vi "Display_ping.vi"(11 "Systèmes inatteignable":string[][](array[string])) -> ()   [LabVIEW 2019]
panel:
  in  "Bouton OK":bool
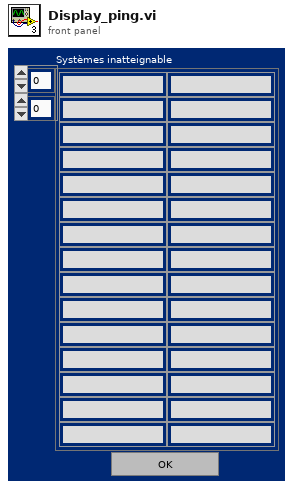
[diagram p1: front panel]
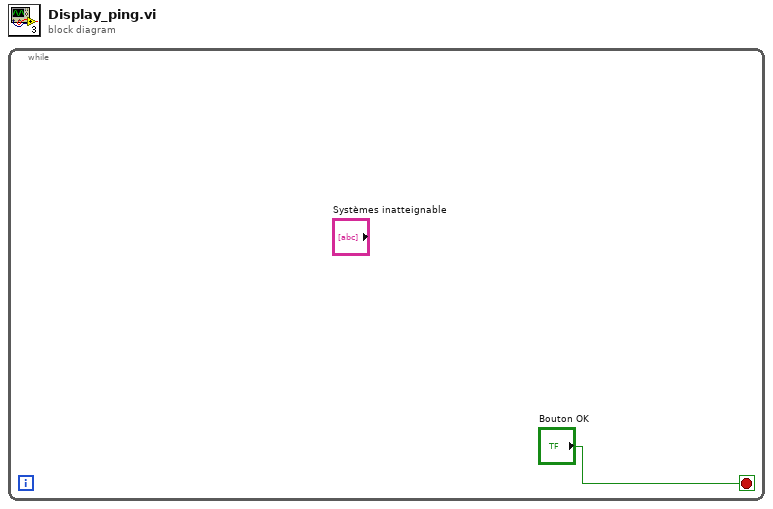
[diagram p0: block diagram]
diagram:
  n1 = while {
    stop <- "Bouton OK" stop-if-true
  }
